vi "Tactic.vi"(0 "points 3":cluster{"x":dbl, "y":dbl}[](array[cluster])=[{"x"=0.0, "y"=0.0}, {"x"=1000.0, "y"=1000.0}, {"x"=-1000.0, "y"=1000.0}], 4 "robot id vel":u32, 6 "atacando ao contrário?":bool=TRUE, 7 "AI Parameters":T1={"GotoKick"={"Dist do cone a frente"=150.0, "attacker farback"=1500.0, "Perto"=300.0, "min dist to kick"=150.0, "kick eps"=0.0, "Time to transition"=0.05}, "Attacker"={"CC chute"=0.09, "CC passe"=0.045, "Kick Force"=100.0, "D ball-robot Kick"=200.0, "D ball-robot Pass"=0.3}, "Defender"={"D max"=1700.0, "Vel p/ robô av"=1000.0, "Kick Force"=100.0, "D atk-def"=0.0, "D farback"=0.0}, "Timeout"={"Field/v in x"=6.0, "Dist Robots"=300, "Dist up in y"=300}, "Pose Striker"={"dist"=200.0, "Numeric"=-4.0, "dist 2"=200.0}, "Dist Stop"=300.0, "Distance when ball out"=200, "D central gap "=150.0, "T pass"=0.0, "Force ++"=0.0, "range kick"=0.0, "Chute alto"=TRUE, "Marcador novo"=TRUE} {"D central gap" format="%#_13g"; "Dist Stop" format="%#_13g"; "Pose Striker"."Numeric" format="%#_13g"; "Defender"."Kick Force" format="%#_13g"; "Defender"."Vel p/ robô av" format="%#_13g"; "Attacker"."D ball-robot Kick" format="%#_13g"; "Attacker"."Kick Force" format="%#_13g"; "Attacker"."CC passe" format="%#_13g"; "Attacker"."CC chute" format="%#_13g"; "GotoKick"."kick eps" format="%#_13g"; "GotoKick"."min dist to kick" format="%#_13g"; "GotoKick"."Perto" format="%#_13g"; "GotoKick"."attacker farback" format="%#_13g"; "GotoKick"."Dist do cone a frente" format="%#_13g"}, 8 "GoTo point":dbl[](array[numeric])=[0.0, 0.0, 0.0], 9 "Defense stretch":i32=600, 10 "Defense radius":i32=400, 11 "IA State Input":T2={"our_robots"=[], "enemy_robots"=[], "balls"=[], "geometry"={"line_width"=0, "field_length"=0, "field_width"=0, "boundary_width"=0, "referee_width"=0, "goal_width"=0, "goal_depth"=0, "goal_wall_width"=0, "center_circle_radius"=0, "defense_radius"=0, "defense_stretch"=0, "free_kick_from_defense_dist"=0, "penalty_spot_from_field_line_dist"=0, "penalty_line_from_spot_dist"=0}, "IA Judge"={"stage"="", "command"="", "our_goalie_id"=0.0, "enemy_goalie_id"=0.0, "command enum"=enum."Halt", "Time"=enum."Azul"}, "Received Timestamp"=timestamp(0 s since 1904-01-01), "Events"={"Touch"=FALSE, "Ball out"=FALSE, "id touch"=0.0, "Ball out of \nVision"=FALSE, "Ball inside \nGoalie area"=FALSE, "Robot not responding"=FALSE, "Robots responding status"=[1.0, 1.0, 1.0, 1.0, 1.0, 1.0], "Enemy Ball \nPossession"=FALSE, "Pass State"=FALSE, "id end of pass"=0.0, "Kick"=FALSE, "Id ini Possession"=0.0, "Ball Possesion"=FALSE, "Id Possesion"=0.0}}) -> (1 "Robot":dbl(graph), 2 "ball":dbl(graph), 3 "IA State Output":T2={"our_robots"=[], "enemy_robots"=[], "balls"=[], "geometry"={"line_width"=0, "field_length"=0, "field_width"=0, "boundary_width"=0, "referee_width"=0, "goal_width"=0, "goal_depth"=0, "goal_wall_width"=0, "center_circle_radius"=0, "defense_radius"=0, "defense_stretch"=0, "free_kick_from_defense_dist"=0, "penalty_spot_from_field_line_dist"=0, "penalty_line_from_spot_dist"=0}, "IA Judge"={"stage"="", "command"="", "our_goalie_id"=0.0, "enemy_goalie_id"=0.0, "command enum"=enum."Halt", "Time"=enum."Azul"}, "Received Timestamp"=timestamp(0 s since 1904-01-01), "Events"={"Touch"=FALSE, "Ball out"=FALSE, "id touch"=0.0, "Ball out of \nVision"=FALSE, "Ball inside \nGoalie area"=FALSE, "Robot not responding"=FALSE, "Robots responding status"=[1.0, 1.0, 1.0, 1.0, 1.0, 1.0], "Enemy Ball \nPossession"=FALSE, "Pass State"=FALSE, "id end of pass"=0.0, "Kick"=FALSE, "Id ini Possession"=0.0, "Ball Possesion"=FALSE, "Id Possesion"=0.0}}, 5 "kick \nerror":dbl)   [LabVIEW 2017]
uses:
  Core/AI Input.ctl
  Core/AI Robot.ctl
  Functions Enum.ctl
  AttackerStates.ctl
  Core/AI Ball.ctl
  Core/Field Size.ctl
  Core/AI Judge.ctl
  Command Enum.ctl
  Util/Events/Events.ctl
  AI Parameters.ctl
  <vilib>/Analysis/_algsub.llb/Real Vector Norm.vi
  <vilib>/Analysis/NI_AALPro.lvlib
panel:
  in  "y":dbl=3000.0 format="%#_13g"
  out "N atacantes":u32[](array[numeric])
  out "Defensores":u32[](array[numeric])
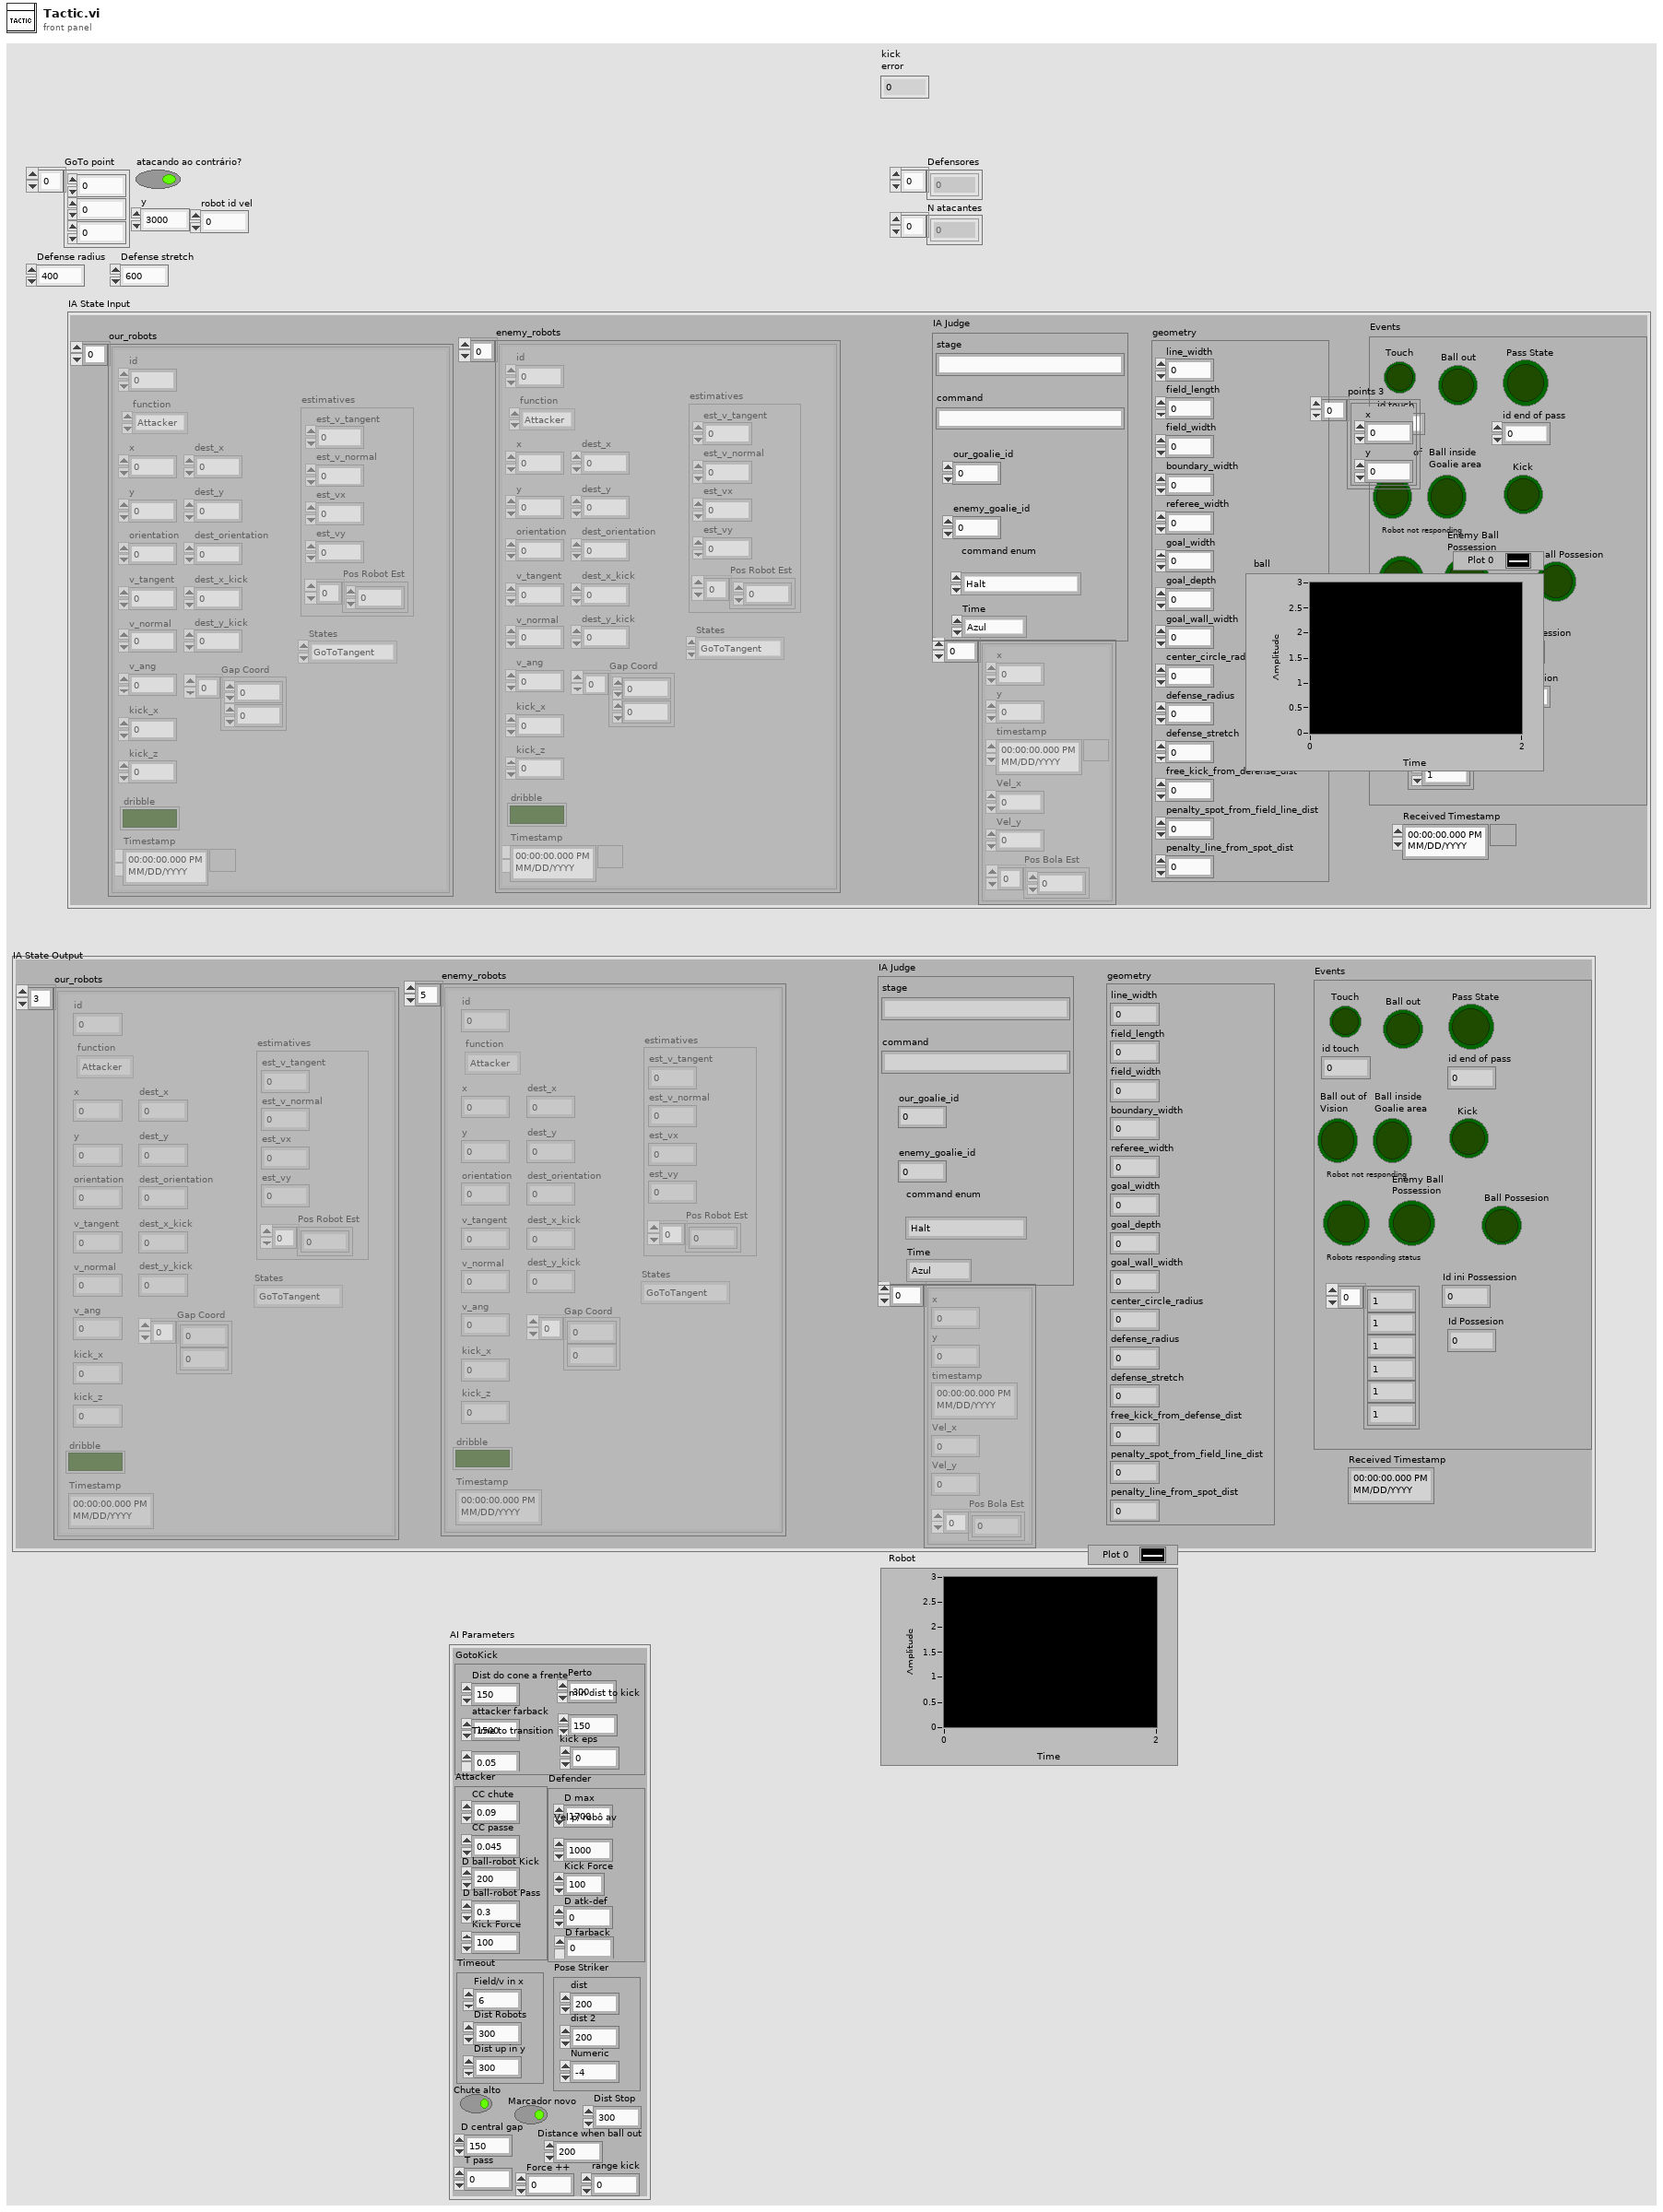
[diagram p1: front panel]
types:
  T1 = typedef "AI Parameters.ctl" = cluster{"GotoKick":cluster{"Dist do cone a frente":dbl, "attacker farback":dbl, "Perto":dbl, "min dist to kick":dbl, "kick eps":dbl, "Time to transition":dbl}, "Attacker":cluster{"CC chute":dbl, "CC passe":dbl, "Kick Force":dbl, "D ball-robot Kick":dbl, "D ball-robot Pass":dbl}, "Defender":cluster{"D max":dbl, "Vel p/ robô av":dbl, "Kick Force":dbl, "D atk-def":dbl, "D farback":dbl}, "Timeout":cluster{"Field/v in x":dbl, "Dist Robots":u32, "Dist up in y":u32}, "Pose Striker":cluster{"dist":dbl, "Numeric":dbl, "dist 2":dbl}, "Dist Stop":dbl, "Distance when ball out":i32, "D central gap ":dbl, "T pass":dbl, "Force ++":dbl, "range kick":dbl, "Chute alto":bool, "Marcador novo":bool}
  T2 = typedef "AI Input.ctl" = cluster{"our_robots":T3[], "enemy_robots":T3[], "balls":T6[], "geometry":T7, "IA Judge":T8, "Received Timestamp":timestamp, "Events":T10}
  T3 = typedef "AI Robot.ctl" = cluster{"id":u32, "function":T4, "x":dbl, "y":dbl, "orientation":dbl, "v_tangent":dbl, "v_normal":dbl, "v_ang":dbl, "kick_x":dbl, "kick_z":dbl, "dribble":bool, "Timestamp":timestamp, "dest_x":dbl, "dest_y":dbl, "dest_orientation":dbl, "estimatives":cluster{"est_v_tangent":dbl, "est_v_normal":dbl, "est_vx":dbl, "est_vy":dbl, "Pos Robot Est":dbl[]}, "dest_x_kick":dbl, "dest_y_kick":dbl, "Gap Coord":dbl[], "States":T5}
  T4 = typedef "Functions Enum.ctl" = enum16{"Attacker", "Goalie", "Defender", "Striker", "Goto 0", "Dummy", "Kicker", "ZigZag"}
  T5 = typedef "AttackerStates.ctl" = enum16{"Pass", "GoToTangent", "BallGetting", "GoToKick", ""}
  T6 = typedef "AI Ball.ctl" = cluster{"x":dbl, "y":dbl, "timestamp":timestamp, "Vel_x":dbl, "Vel_y":dbl, "Pos Bola Est":dbl[]}
  T7 = typedef "Field Size.ctl" = cluster{"line_width":u32, "field_length":u32, "field_width":u32, "boundary_width":u32, "referee_width":u32, "goal_width":u32, "goal_depth":u32, "goal_wall_width":u32, "center_circle_radius":u32, "defense_radius":u32, "defense_stretch":u32, "free_kick_from_defense_dist":u32, "penalty_spot_from_field_line_dist":u32, "penalty_line_from_spot_dist":u32}
  T8 = typedef "AI Judge.ctl" = cluster{"stage":string, "command":string, "our_goalie_id":dbl, "enemy_goalie_id":dbl, "command enum":T9, "Time":enum16{"Azul", "Amarelo"}}
  T9 = typedef "Command Enum.ctl" = enum16{"Halt", "Stop", "Force Start", "PKA Normal Start", "Prepare Kickoff Ally", "PKE Normal Start", "Prepare Kickoff Enemy", "Prepare Penalty Ally", "PPA Normal Start", "Prepare Penalty Enemy", "PPE Normal Start", "Direct Free Enemy", "Direct Free Ally", "Indirect Free Enemy", "Indirect Free Ally", "Timeout Enemy", "Timeout Ally", "Goal Enemy", "Goal Ally", "Ball Placement Enemy", "Ball Placement Ally", "Normal Half Time", "Extra Time Break", "Extra Half Time", "None", "Post Game"}
  T10 = typedef "Events.ctl" = cluster{"Touch":bool, "Ball out":bool, "id touch":dbl, "Ball out of \nVision":bool, "Ball inside \nGoalie area":bool, "Robot not responding":bool, "Robots responding status":dbl[], "Enemy Ball \nPossession":bool, "Pass State":bool, "id end of pass":dbl, "Kick":bool, "Id ini Possession":dbl, "Ball Possesion":bool, "Id Possesion":dbl}
  T11 = cluster{"est_v_tangent":dbl, "est_v_normal":dbl, "est_vx":dbl, "est_vy":dbl, "Pos Robot Est":dbl[]}
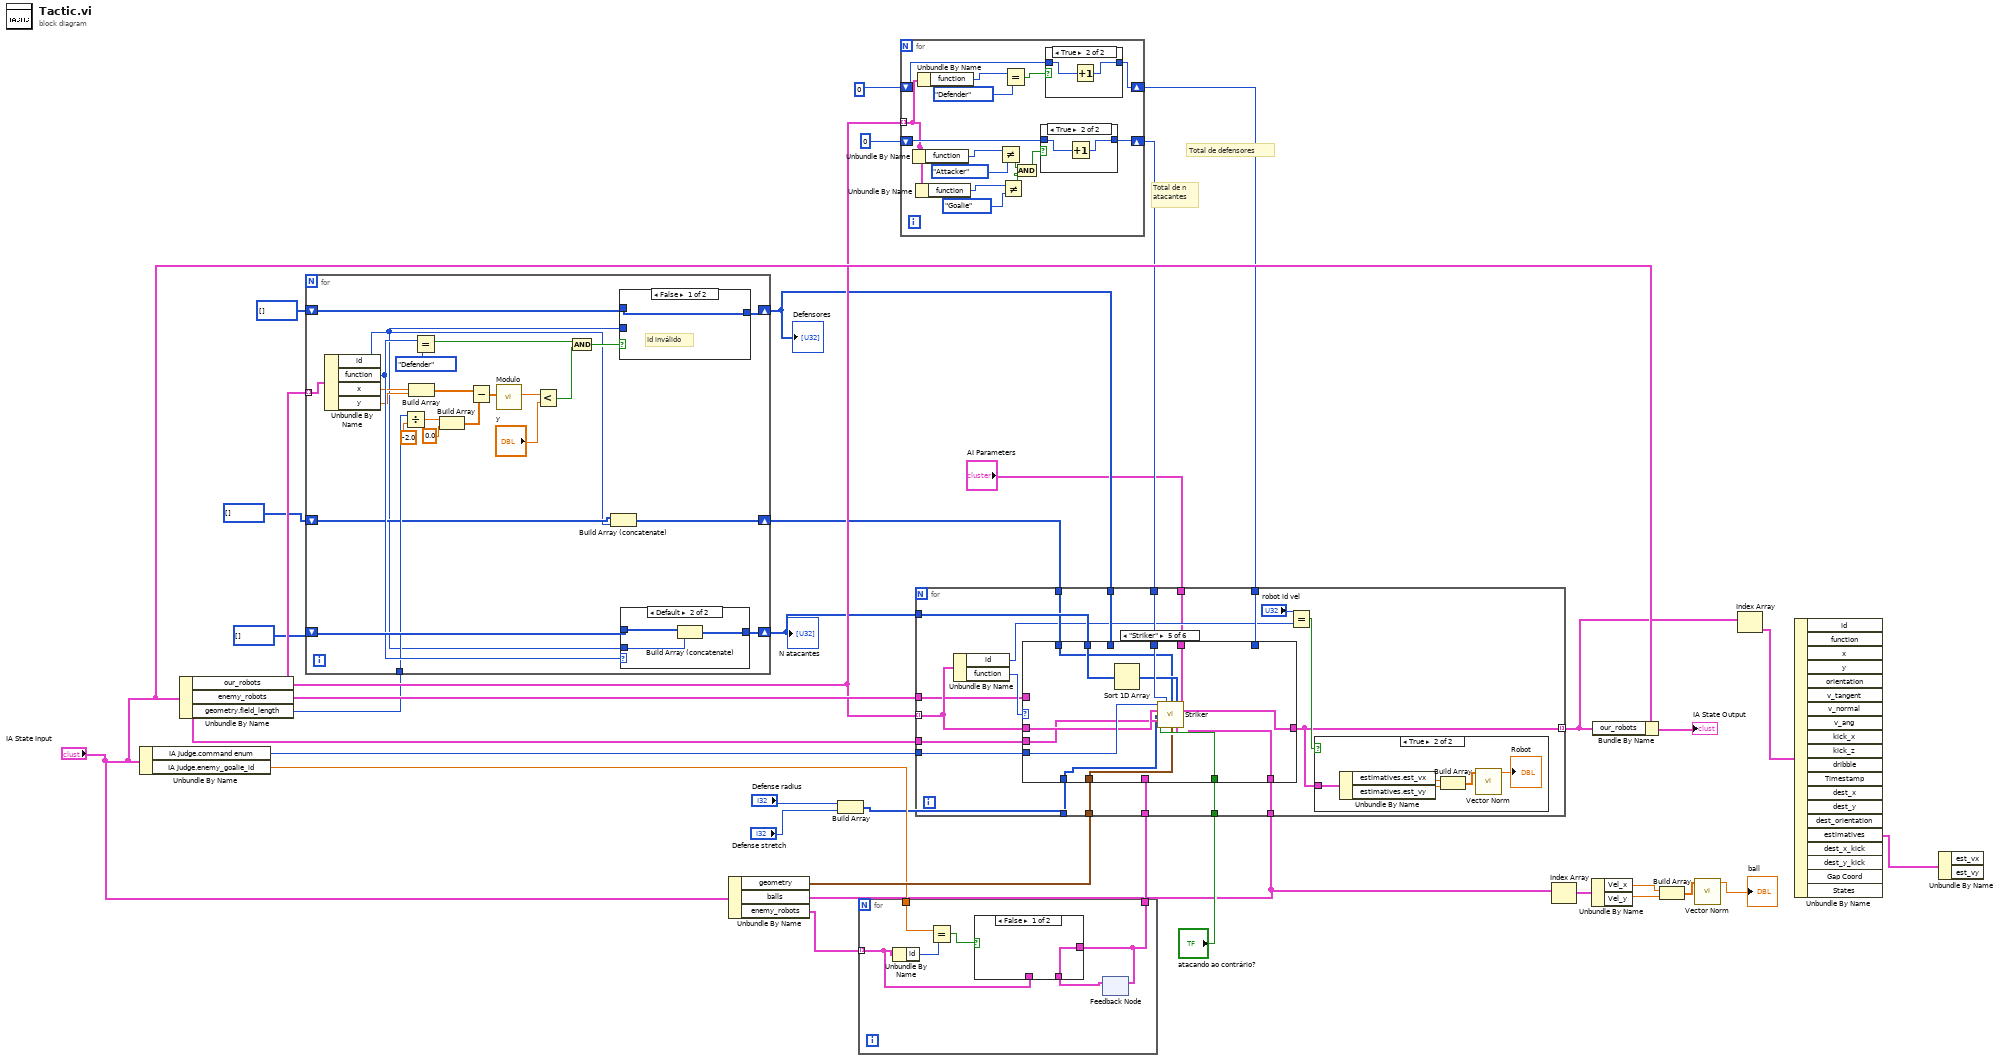
[diagram p0: block diagram]
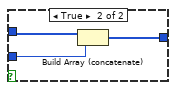
[diagram p3: hidden frame]
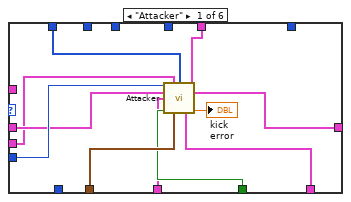
[diagram p8: hidden frame]
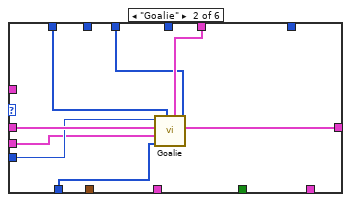
[diagram p9: hidden frame]
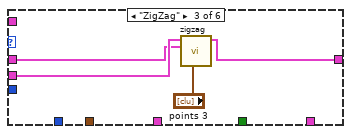
[diagram p10: hidden frame]
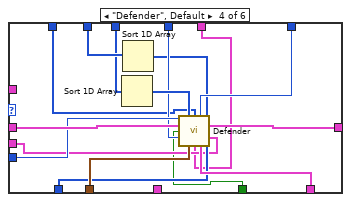
[diagram p11: hidden frame]
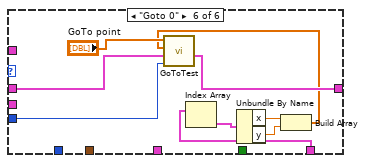
[diagram p12: hidden frame]
diagram:
  # "Total de n\natacantes"
  # "Total de defensores"
  n1 = Unbundle By Name("IA State Input") -> ("IA Judge.command enum"=w34:T9, "IA Judge.enemy_goalie_id"=w28:dbl)
  n2 = Unbundle By Name("IA State Input") -> ("our_robots"=w23:T3[], "enemy_robots"=w25:T3[], "geometry.field_length"=w13:u32)
  n3 = for {
    tunnel: w23 -> [w58] mode=indexing
    shift-right: [w57] -> w14
    shift-left: u32[] [] -> [w55]
    shift-right: [w56] -> w15
    shift-left: u32[] [] -> [w54]
    tunnel: w13 -> [w49]
    shift-right: [w35] -> w5
    shift-left: u32[] [] -> [w37]
    n4 = Unbundle By Name(w58) -> ("id"=w36:u32, "function"=w53:T4, "x"=w51:dbl, "y"=w50:dbl)
    n5 = Divide(x=w49, y=-2.0) -> (x/y=w47:dbl)
    n6 = Build Array(w51, w50) -> (w44:dbl[])
    n7 = Equal?(x=w53, y=Functions_Enum."Defender" ("function")) -> (x = y?=w38:bool)
    n8 = Build Array(w47, 0.0 ("element")) -> (w45:dbl[])
    n9 = Subtract(x=w44, y=w45) -> (x-y=w43:dbl[])
    n10 = call "Modulo.vi"("2D vector"=w43) -> ("Modulo"=w42:dbl)  [unwired: 10 in]
    n11 = Less?(x=w42, y="y") -> (x < y?=w39:bool)
    n12 = And(x=w38, y=w39) -> (x .and. y?=w40:bool)
    n13 = Build Array (concatenate)(w37, w36) -> (w35:u32[])
    n14 = case shown="False" w40 {
      tunnel: w36 -> [_ w66]
      tunnel: w55 -> [w63 w65]
      tunnel: [w63 w64] -> w57
      frame False {
        # "Id inválido"
      }
      frame True {
        n15 = Build Array (concatenate)(w65, w66) -> (w64:u32[])
      }
    }
    n16 = case shown="Default" w53 {
      tunnel: w36 -> [_ w62]
      tunnel: w54 -> [w59 w61]
      tunnel: [w59 w60] -> w56
      frame "Attacker", "Goalie" {
        # "Id inválido"
      }
      frame Default {
        n17 = Build Array (concatenate)(w61, w62) -> (w60:u32[])
      }
    }
  }
  "Defensores" <- w14
  "N atacantes" <- w15
  n18 = Unbundle By Name("IA State Input") -> ("geometry"=w31:T7, "balls"=w7:T6[], "enemy_robots"=w30:T3[])
  n19 = Build Array("Defense radius", "Defense stretch") -> (w16:i32[])
  n20 = for {
    tunnel: w30 -> [w69] mode=indexing
    tunnel: [w68] -> w29
    tunnel: w28 -> [w72]
    n21 = Unbundle By Name(w69) -> ("id"=w71:u32)
    n22 = Equal?(x=w72, y=w71) -> (x = y?=w70:bool)
    n23 = feedback #1() -> (w67:T3)  [unwired: 1 in]
    n24 = case shown="False" w70 {
      tunnel: w69 -> [_ w74]
      tunnel: [w73 w74] -> w68
      tunnel: w67 -> [w73 _]
      frame False {
      }
      frame True {
      }
    }
    n25 = feedback-in #1(w68) -> ()
  }
  n26 = for {
    tunnel: w23 -> [w80] mode=indexing
    shift-right: [w85] -> w26
    shift-left: 0 -> [w86]
    shift-right: [w81] -> w20
    shift-left: 0 -> [w82]
    n27 = Unbundle By Name(w80) -> ("function"=w84:T4)
    n28 = Unbundle By Name(w80) -> ("function"=w75:T4)
    n29 = Unbundle By Name(w80) -> ("function"=w89:T4)
    n30 = Not Equal?(x=w84, y=Functions_Enum."Attacker") -> (x != y?=w78:bool)
    n31 = Not Equal?(x=w75, y=Functions_Enum."Goalie") -> (x != y?=w79:bool)
    n32 = Equal?(x=w89, y=Functions_Enum."Defender") -> (x = y?=w87:bool)
    n33 = And(x=w78, y=w79) -> (x .and. y?=w77:bool)
    n34 = case shown="True" w77 {
      tunnel: w82 -> [w90 w92]
      tunnel: [w90 w91] -> w81
      frame False {
      }
      frame True {
        n35 = Increment(x=w92) -> (x+1=w91:i32)
      }
    }
    n36 = case shown="True" w87 {
      tunnel: w86 -> [w93 w95]
      tunnel: [w93 w94] -> w85
      frame False {
      }
      frame True {
        n37 = Increment(x=w95) -> (x+1=w94:i32)
      }
    }
  }
  n38 = for {
    tunnel: w23 -> [w114] mode=indexing
    tunnel: [w97] -> w3 mode=indexing
    tunnel: w34 -> [w113]
    tunnel: "IA State Input" -> [w112]
    tunnel: w31 -> [w111]
    tunnel: w7 -> [w110]
    tunnel: w29 -> [w109]
    tunnel: w26 -> [w108]
    tunnel: w25 -> [w107]
    tunnel: "atacando ao contrário?" -> [w106]
    tunnel: w20 -> [w105]
    tunnel: w16 -> [w104]
    tunnel: w15 -> [w103]
    tunnel: w14 -> [w102]
    tunnel: w5 -> [w101]
    tunnel: "AI Parameters" -> [w96]
    n39 = Unbundle By Name(w114) -> ("id"=w99:u32, "function"=w115:T4)
    n40 = case shown="\"Striker\"" w115 {
      tunnel: w114 -> [w125 w139 w141 w159 w171 w180]
      tunnel: [w131 w138 w143 w157 w166 w179] -> w97
      tunnel: w113 -> [w130 w137 _ w158 w172 w178]
      tunnel: w112 -> [w124 w136 w142 w147 w170 _]
      tunnel: w111 -> [w129 _ _ w156 w167 _]
      tunnel: w110 -> [w128 _ _ w155 w168 w177]
      tunnel: w109 -> [w126 _ _ _ _ _]
      tunnel: w108 -> [_ _ _ w154 _ _]
      tunnel: w107 -> [_ _ _ _ _ _]
      tunnel: w106 -> [w127 _ _ w144 w169 _]
      tunnel: w105 -> [_ _ _ w152 w165 _]
      tunnel: w104 -> [_ w135 _ w150 w160 _]
      tunnel: w103 -> [_ _ _ w149 w163 _]
      tunnel: w102 -> [_ w132 _ w148 _ _]
      tunnel: w101 -> [w123 w134 _ w146 w162 _]
      tunnel: w96 -> [w122 w133 _ w145 w161 _]
      frame "Attacker" {
        n41 = call "Attacker.vi"("command\nenum"=w130, "IA State Input 2"=w124, "Total de robos"=w123, "AI Parameters"=w122, "Robot in"=w125, "Opponent goalie"=w126, "atacando contra?"=w127, "Field Size 2"=w129, "balls"=w128) -> ("output cluster"=w131:T3, "kick \nerror"=→"kick \nerror":dbl)  [unwired: 5 in]
      }
      frame "Goalie" {
        n42 = call "Goalie.vi"("Defensores"=w132, "AI Parameters"=w133, "Total de robos"=w134, "Field defense"=w135, "IA Input"=w136, "Robot"=w139, "command\nenum"=w137) -> ("output cluster"=w138:T3)  [unwired: 4 in]
      }
      frame "ZigZag" {
        n43 = call "zigzag.vi"("points 3"="points 3", "Current Robot"=w141, "Al Input"=w142) -> ("Output Robot"=w143:T3)  [unwired: 8 in]
      }
      frame "Defender", Default {
        n44 = Sort 1D Array(array=w148) -> (sorted array=w153:u32[])
        n45 = Sort 1D Array(array=w149) -> (sorted array=w151:u32[])
        n46 = call "Defender.vi"("command\nenum"=w158, "Defensores"=w153, "Total de robos"=w146, "total de \ndefensores"=w154, "N atacantes"=w151, "Our Robots"=w159, "Atacando contra?"=w144, "Total de n\natacantes"=w152, "IA State Input 2"=w147, "Field Size 2"=w156, "AI Parameters"=w145, "balls"=w155, "Field defense"=w150) -> ("output cluster"=w157:T3)  [unwired: 2 in]
      }
      frame "Striker" {
        n47 = Sort 1D Array(array=w163) -> (sorted array=w164:u32[])
        n48 = call "Striker.vi"("command\nenum"=w172, "Toral de n\natacantes"=w165, "Total de robos"=w162, "N atacantes"=w164, "AI Parameters"=w161, "Robot"=w171, "Field defense"=w160, "IA Input"=w170, "atacando ao contrário?"=w169, "Field Size 2"=w167, "balls"=w168) -> ("Robot out"=w166:T3)  [unwired: 4 in]
      }
      frame "Goto 0" {
        n49 = Index Array(array=w177) -> (element=w176:T6)  [unwired: 1 in]
        n50 = Unbundle By Name(w176) -> ("x"=w175:dbl, "y"=w174:dbl)
        n51 = Build Array(w175, w174) -> (w173:dbl[])
        n52 = call "GoToTest.vi"("command\nenum"=w178, "Robot In"=w180, "Ball"=w173, "GoTo point"="GoTo point") -> ("Robot Out"=w179:T3)  [unwired: 7 in]
      }
    }
    n53 = Equal?(x="robot id vel", y=w99) -> (x = y?=w98:bool)
    n54 = case shown="True" w98 {
      tunnel: w97 -> [_ w116]
      frame False {
      }
      frame True {
        n55 = Unbundle By Name(w116) -> ("estimatives.est_vx"=w120:dbl, "estimatives.est_vy"=w119:dbl)
        n56 = Build Array(w120, w119) -> (w118:dbl[])
        n57 = call-poly <vilib>:"Vector Norm.vi"("Input Vector"=w118) -> ("norm"=→"Robot":dbl)  [unwired: 9 in, 1 out]
      }
    }
  }
  n58 = Index Array(array=w7) -> (element=w12:T6)  [unwired: 1 in]
  n59 = Unbundle By Name(w12) -> ("Vel_x"=w10:dbl, "Vel_y"=w9:dbl)
  n60 = Bundle By Name(cluster="IA State Input", "our_robots"=w3) -> (→"IA State Output":T2)
  n61 = Build Array(w10, w9) -> (w11:dbl[])
  n62 = call-poly <vilib>:"Vector Norm.vi"("Input Vector"=w11) -> ("norm"=→"ball":dbl)  [unwired: 9 in, 1 out]
  n63 = Index Array(array=w3) -> (element=w2:T3)  [unwired: 1 in]
  n64 = Unbundle By Name(w2) -> ("estimatives"=w1:T11)  [unwired: 19 out]
  n65 = Unbundle By Name(w1) -> ()  [unwired: 2 out]
